vi "Write Double.vi"(8 "error in (no error)":errorcluster, 10 "value":dbl, 11 "DataSingleElement in":refnum<class "DataSingleElement.lvclass">) -> (0 "error out":errorcluster, 3 "DataSingleElement out":refnum<class "DataSingleElement.lvclass">)   [LabVIEW 2014, in "DataSingleElement.lvclass"]
uses:
  DataSingleElement.lvclass
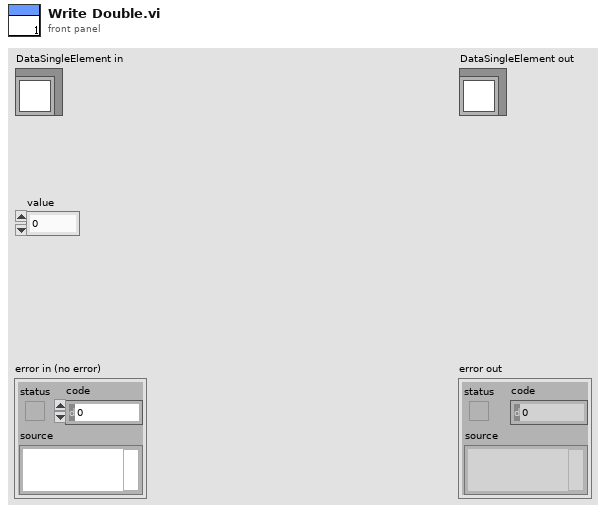
[diagram p1: front panel]
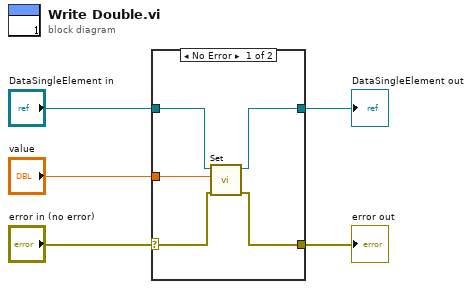
[diagram p0: block diagram]
diagram:
  n1 = case shown="No Error" "error in (no error)" {
    selector: "error in (no error)" -> [w7 w12]
    tunnel: [w6 w12] -> w4
    tunnel: [w8 w11] -> w2
    tunnel: "DataSingleElement in" -> [w9 w11]
    tunnel: "value" -> [w10 _]
    frame No Error {
      n2 = call-dynamic "Set.vi"("error in (no error)"=w7, "Data"=w10, "AbstractData in"=w9) -> ("error out"=w6:errorcluster, "AbstractData out"=w8:refnum<class "DataSingleElement.lvclass">)  [unwired: 7 in]
    }
    frame Error {
    }
  }
  "error out" <- w4
  "DataSingleElement out" <- w2
